vi "DJ Boczko.vi"(5 "TRUE = Hora Local\nFALSE = UT":bool) -> (1 "ANO":i32, 2 "MES":i32, 3 "DIA":i32, 4 "hour":i32, 6 "minute":i32, 8 "second":i32, 10 "Dia Juliano":dbl format="%.8f", 14 "Dia Juliano Inteiro":dbl, 15 "Dia Juliano Modificado":dbl format="%.8f")   [LabVIEW 2018]
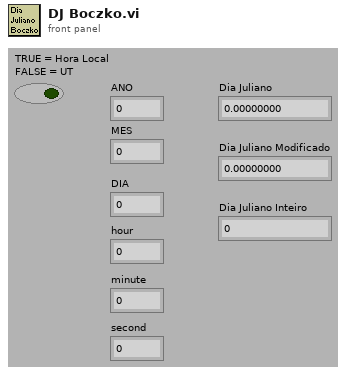
[diagram p1: front panel]
types:
  T1 = cluster{"second":i32, "minute":i32, "hour":i32, "day of month":i32, "month":i32, "year":i32, "day of week":i32, "day of year":i32, "is DST":i32}
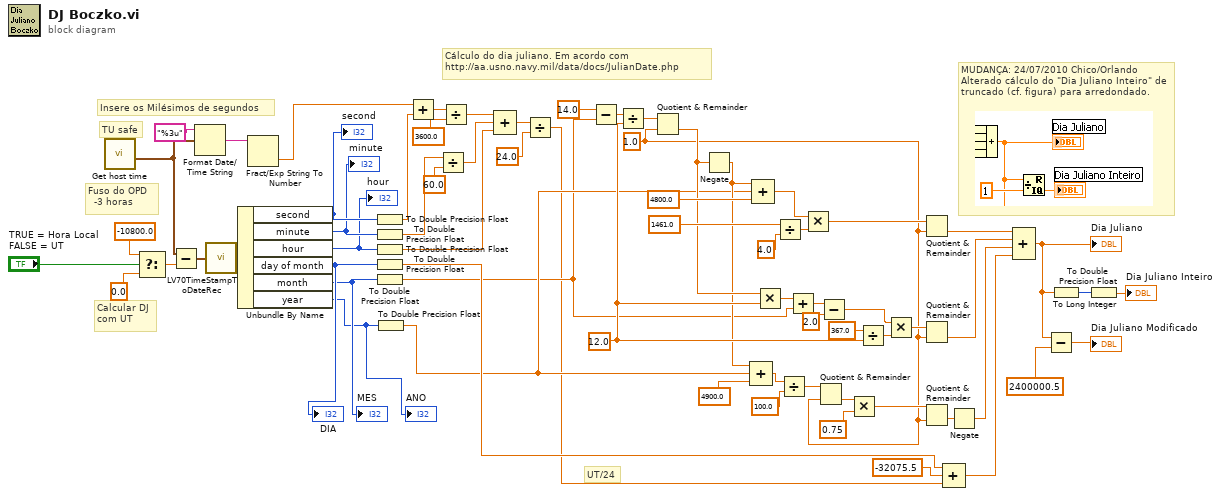
[diagram p0: block diagram]
diagram:
  w17 = 1.0 ("y")
  w53 = 12.0 ("y")
  # "TU safe"
  # "MUDANÇA: 24/07/2010 Chico/Orlando\nAlterado cálculo do \"Dia Juliano Inteiro\" de truncado (cf. figura) para arredondado."
  # "Calcular DJ\ncom UT"
  # "Fuso do OPD\n  -3 horas"
  # "Insere os Milésimos de segundos"
  # "UT/24"
  # "Cálculo do dia juliano. Em acordo com \nhttp://aa.usno.navy.mil/data/docs/JulianDate.php"
  n1 = call "Get host time.vi"() -> ("BR current time"=w1:timestamp)  [unwired: 8 in, 3 out]
  n2 = Select(t=-10800.0 ("Fuso"), s="TRUE = Hora Local\nFALSE = UT", f=0.0 ("Fuso")) -> (s? t:f=w5:dbl)
  n3 = Subtract(x=w1, y=w5) -> (x-y=w18:timestamp)
  n4 = Format Date/Time String(time format string (%c)="%3u", seconds (now)=w1) -> (date/time string=w12:string)  [unwired: 1 in]
  n5 = call <vilib>:"LV70TimeStampToDateRec.vi"("time stamp"=w18) -> ("date time rec"=w36:T1)
  n6 = Unbundle By Name(w36) -> ("second"=w35:i32, "minute"=w34:i32, "hour"=w33:i32, "day of month"=w16:i32, "month"=w15:i32, "year"=w14:i32)
  "ANO" <- w14
  "MES" <- w15
  "DIA" <- w16
  "second" <- w35
  "minute" <- w34
  "hour" <- w33
  n7 = Fract/Exp String To Number(string=w12) -> (number=w11:dbl)  [unwired: 3 in, 1 out]
  n8 = To Double Precision Float(number=w35) -> (double precision float=w9:dbl)
  n9 = To Double Precision Float(number=w34) -> (double precision float=w30:dbl)
  n10 = To Double Precision Float(number=w33) -> (double precision float=w27:dbl)
  n11 = To Double Precision Float(number=w16) -> (double precision float=w26:dbl)
  n12 = To Double Precision Float(number=w15) -> (double precision float=w24:dbl)
  n13 = To Double Precision Float(number=w14) -> (double precision float=w25:dbl)
  n14 = Add(x=w11, y=w9) -> (x+y=w10:dbl)
  n15 = Divide(x=w30, y=60.0) -> (x/y=w28:dbl)
  n16 = Divide(x=w10, y=3600.0) -> (x/y=w29:dbl)
  n17 = Compound Arithmetic op=ADD(w29, w28, w27) -> (w22:dbl)
  n18 = Divide(x=w22, y=24.0) -> (x/y=w21:dbl)
  n19 = Subtract(x=14.0, y=w24) -> (x-y=w67:dbl)
  n20 = Divide(x=w67, y=w53) -> (x/y=w66:dbl)
  n21 = Quotient & Remainder(x=w66, y=w17) -> (floor(x/y)=w60:dbl)  [unwired: 1 out]
  n22 = Negate(x=w60) -> (-x=w49:dbl)
  n23 = Compound Arithmetic op=ADD(w49, w25, 4900.0 ("value")) -> (w47:dbl)
  n24 = Compound Arithmetic op=ADD(w49, w25, 4800.0 ("value")) -> (w61:dbl)
  n25 = Multiply(x=w60, y=w53) -> (x*y=w59:dbl)
  n26 = Divide(x=1461.0, y=4.0) -> (x/y=w62:dbl)
  n27 = Divide(x=w47, y=100.0) -> (x/y=w46:dbl)
  n28 = Add(x=w59, y=w24) -> (x+y=w58:dbl)
  n29 = Multiply(x=w61, y=w62) -> (x*y=w52:dbl)
  n30 = Quotient & Remainder(x=w46, y=w17) -> (floor(x/y)=w45:dbl)  [unwired: 1 out]
  n31 = Subtract(x=w58, y=2.0) -> (x-y=w54:dbl)
  n32 = Multiply(x=w45, y=0.75 ("x")) -> (x*y=w42:dbl)
  n33 = Divide(x=367.0, y=w53) -> (x/y=w56:dbl)
  n34 = Multiply(x=w54, y=w56) -> (x*y=w51:dbl)
  n35 = Quotient & Remainder(x=w52, y=w17) -> (floor(x/y)=w40:dbl)  [unwired: 1 out]
  n36 = Quotient & Remainder(x=w51, y=w17) -> (floor(x/y)=w39:dbl)  [unwired: 1 out]
  n37 = Quotient & Remainder(x=w42, y=w17) -> (floor(x/y)=w43:dbl)  [unwired: 1 out]
  n38 = Compound Arithmetic op=ADD(w26, -32075.5 ("value"), w21) -> (w37:dbl)
  n39 = Negate(x=w43) -> (-x=w38:dbl)
  n40 = Compound Arithmetic op=ADD(w40, w39, w38, w37) -> (w4:dbl)
  "Dia Juliano" <- w4
  n41 = Subtract(x=w4, y=2400000.5) -> (x-y=→"Dia Juliano Modificado":dbl)
  n42 = To Long Integer(number=w4) -> (32bit integer=w3:i32)
  n43 = To Double Precision Float(number=w3) -> (double precision float=→"Dia Juliano Inteiro":dbl)
